vi "SetAngleCruz.vi"(1 "Time Acceleration":dbl, 2 "Angular Velocity":dbl, 3 "Time Manager Output":dbl) -> (0 "Current Angle":dbl)   [LabVIEW 2015]
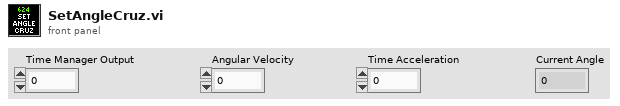
[diagram p1: front panel]
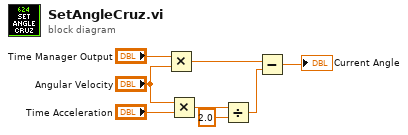
[diagram p0: block diagram]
diagram:
  n1 = Multiply(x="Time Manager Output", y="Angular Velocity") -> (x*y=w3:dbl)
  n2 = Multiply(x="Angular Velocity", y="Time Acceleration") -> (x*y=w5:dbl)
  n3 = Divide(x=w5, y=2.0 ("x")) -> (x/y=w2:dbl)
  n4 = Subtract(x=w3, y=w2) -> (x-y=→"Current Angle":dbl)
